vi "Lay an Egg.vi"(8 "error in (no error)":errorcluster, 11 "Chicken in":refnum<class "Chicken.lvclass">) -> (0 "error out":errorcluster, 3 "Chicken out":refnum<class "Chicken.lvclass">)   [LabVIEW 2024, in "Chicken.lvclass"]
doc: "本VI是为《我和LabVIEW》一书编写的示例。\n关于本书的介绍请参考网页：\nhttp://ruanqizhen.spaces.live.com/blog/cns!5852D4F797C53FB6!4310.entry"
uses:
  Chicken.lvclass
  Chicken.lvclass/Chicken.ctl
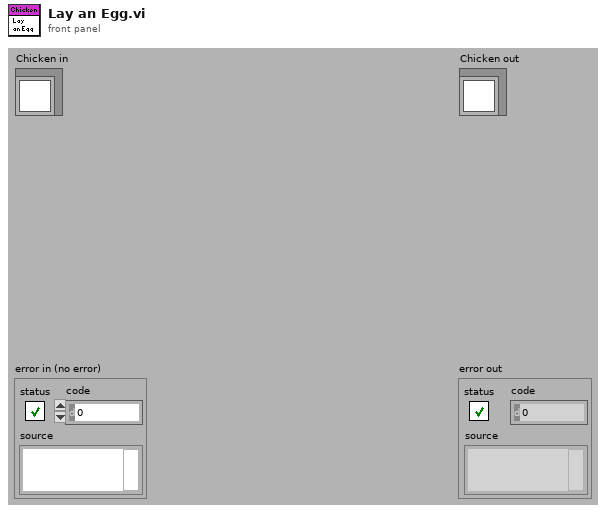
[diagram p1: front panel]
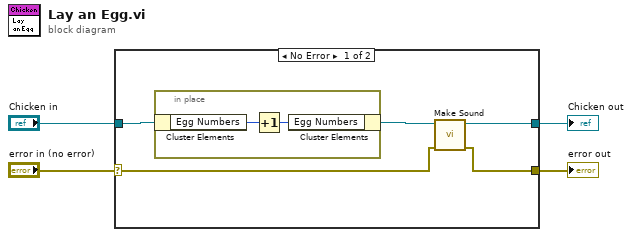
[diagram p0: block diagram]
diagram:
  n1 = case shown="No Error" "error in (no error)" {
    selector: "error in (no error)" -> [w6 w13]
    tunnel: [w5 w13] -> w3
    tunnel: [w7 w12] -> w1
    tunnel: "Chicken in" -> [w8 w12]
    frame No Error {
      n2 = in-place {
        n3 = in-place-cluster #1(w8) -> ("Egg Numbers"=w11:u32)
        n4 = Increment(x=w11) -> (x+1=w10:u32)
        n5 = in-place-cluster #1("Egg Numbers"=w10) -> (w9:refnum<class "Chicken.lvclass">)
      }
      n6 = call-dynamic "Make Sound.vi"("error in (no error)"=w6, "Chicken in"=w9) -> ("error out"=w5:errorcluster, "Chicken out"=w7:refnum<class "Chicken.lvclass">)  [unwired: 8 out]
    }
    frame Error {
    }
  }
  "error out" <- w3
  "Chicken out" <- w1
